vi "CSEI_log.vi"() -> ()   [LabVIEW 2010]
uses:
  <vilib>/Platform/TimedLoop/XDataNode/wakeup.ctl
  <vilib>/Platform/TimedLoop/XDataNode/XDNodeRunTimeDep.lvlib
  <vilib>/Platform/TimedLoop/XDataNode/nitl_modes.ctl
  <vilib>/Platform/TimedLoop/XDataNode/timing_clust.ctl
  <vilib>/Platform/TimedLoop/XDataNode/XDataNode.xnode
panel:
  out "Sample #":dbl
  out "Elapsed Time [s]":dbl
  out "Write to file":string
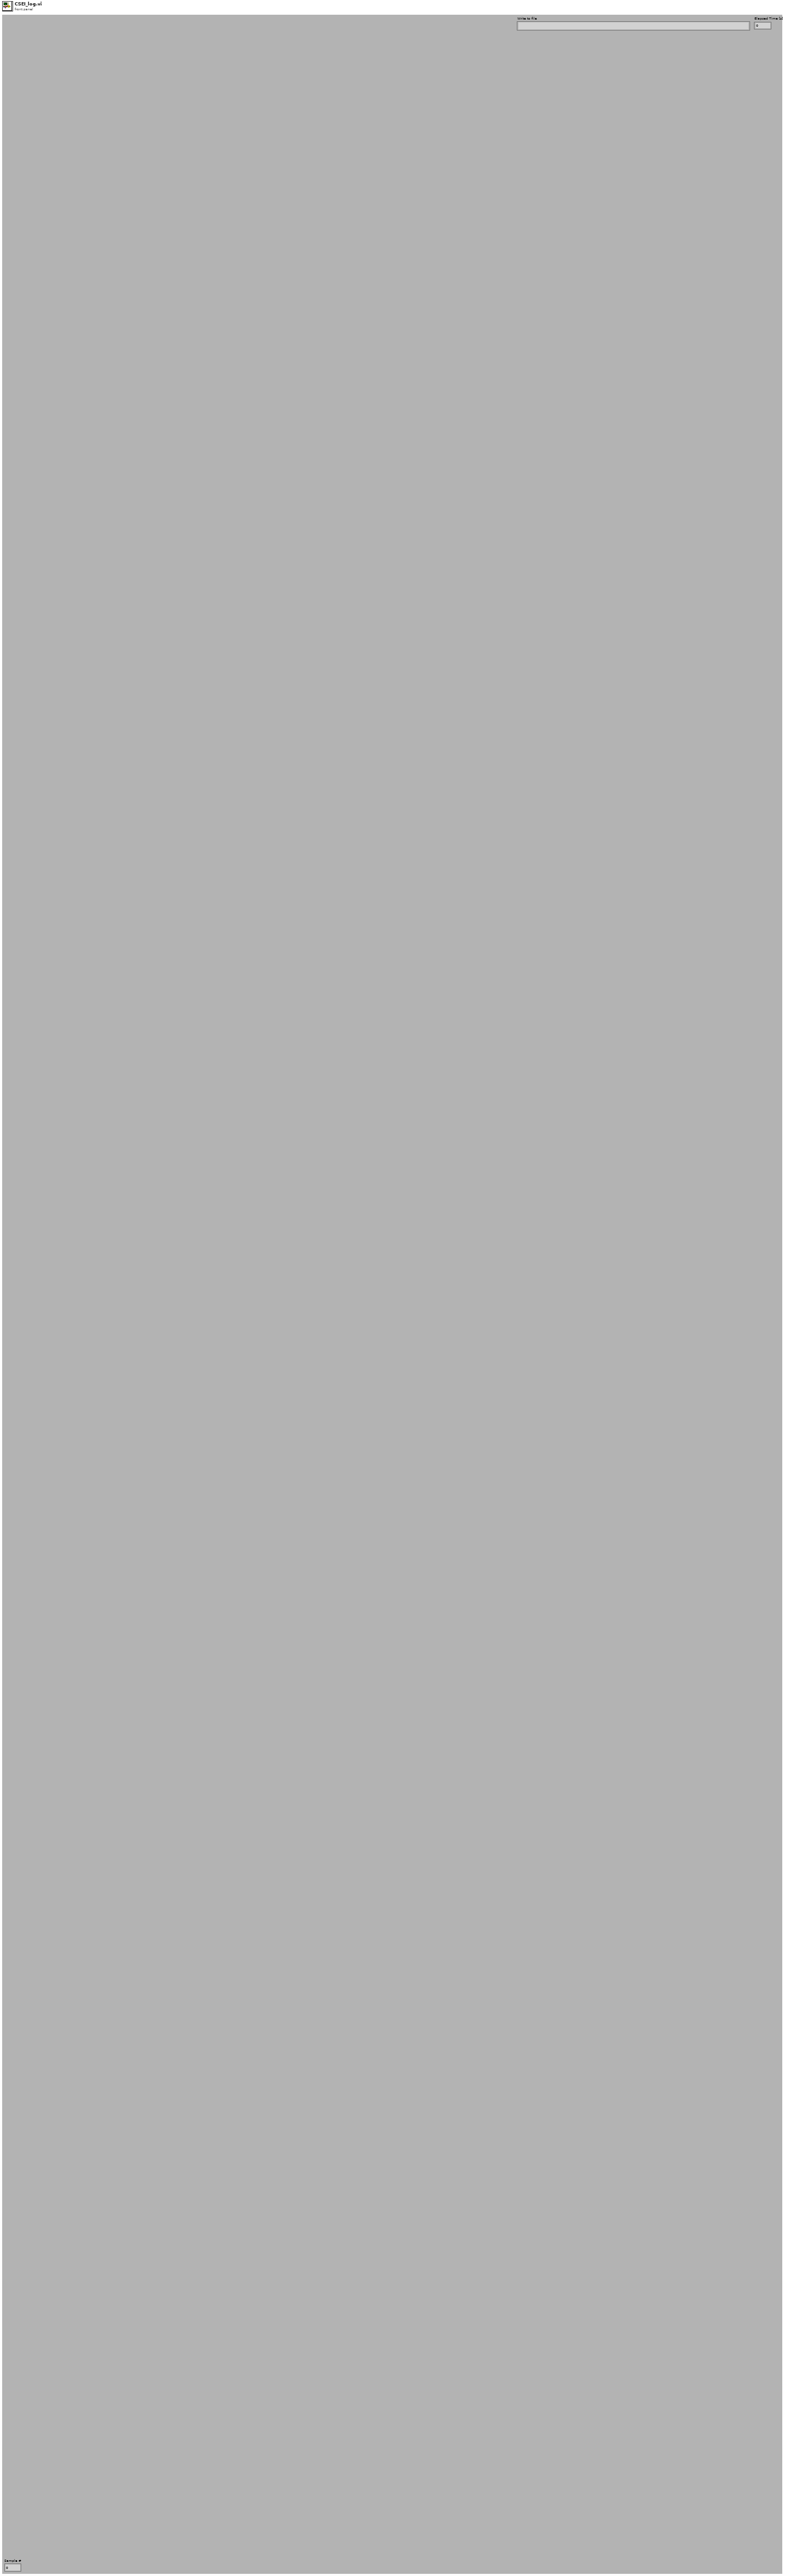
[diagram p1: front panel]
types:
  T1 = enum16{"open", "replace", "create", "open or create", "replace or create", "replace or create with confirmation"}
  T2 = typedef "XDNodeRunTimeDep.lvlib/timing_clust.ctl" = cluster{"Expected End [f-1]":u64, "Actual End [f-1]":u64, "Finished Late? [f-1]":bool, "Expected End [i-1]":u64, "Actual End [i-1]":u64, "Finished Late? [i-1]":bool, "Expected Start [i]":u64, "Actual Start [i]":u64, "Expected Start [f]":u64, "Actual Start [f]":u64, "Source Name":string, "Structure Name":string, "Period":i64, "Deadline":i64, "Offset":i64, "Start":i64, "Priority":i32, "Timeout":i32, "Mode":T3, "Wakeup Reason":T4, "Error":errorcluster, "Source Type":string, "Secondary Source Type":string, "Global End Time":u64, "Global Start Time":u64, "Frame Duration":u64, "Iteration Duration":u64, "Assigned CPU":i32, "I/O Scan Engine Mode":u32}
  T3 = typedef "XDNodeRunTimeDep.lvlib/nitl_modes.ctl" = enum32{"No Change", "Process missed periods, maintain original phase", "Discard missed periods, maintain original phase", "Process missed periods, ignore original phase", "Discard missed periods, ignore original phase"}
  T4 = typedef "XDNodeRunTimeDep.lvlib/wakeup.ctl" = enum32{"Normal", "Aborted", "Asynchronous wakeup", "Timing source error", "Timed loop error", "Timeout"}
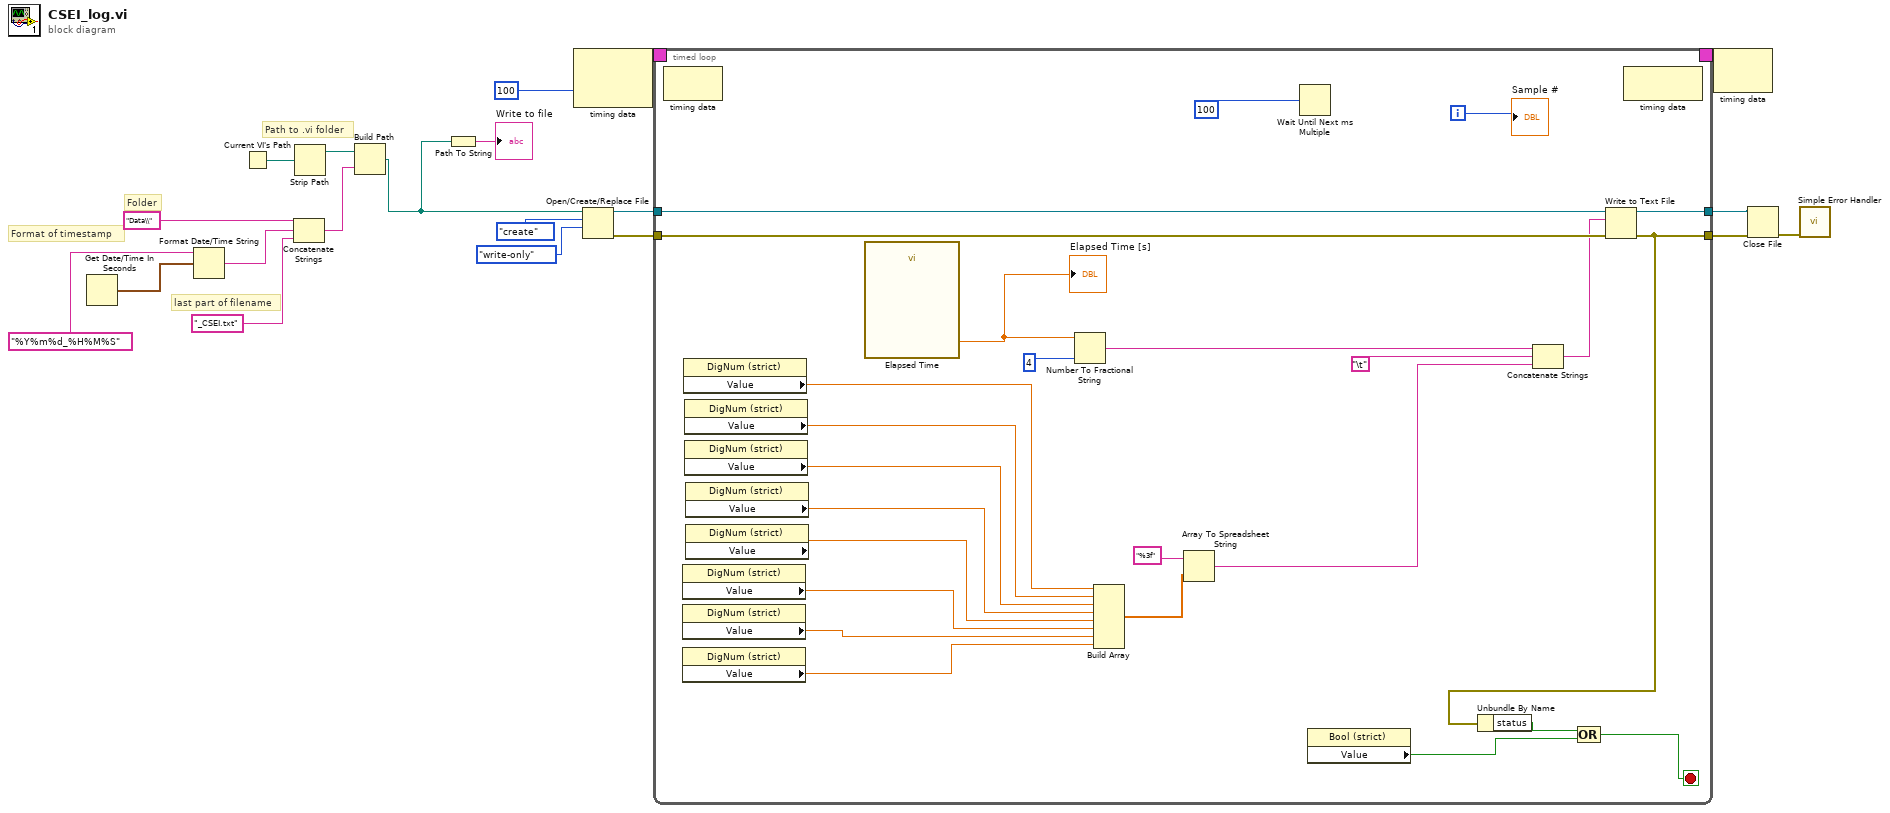
[diagram p0: block diagram]
diagram:
  # "Path to .vi folder"
  # "last part of filename"
  # "Folder"
  # "Format of timestamp"
  n1 = Get Date/Time In Seconds() -> (seconds since 1Jan1904=w17:timestamp)
  n2 = Format Date/Time String(time format string (%c)="%Y%m%d_%H%M%S", seconds (now)=w17) -> (date/time string=w15:string)  [unwired: 1 out]
  n3 = Current VI's Path() -> (path=w1:path)
  n4 = Concatenate Strings("Data\\" ("string"), w15, "_CSEI.txt" ("string")) -> (w12:string)
  n5 = Strip Path(path=w1) -> (stripped path=w14:path)  [unwired: 1 out]
  n6 = Build Path(base path=w14, name or relative path=w12) -> (appended path=w8:path)
  n7 = Path To String(path=w8) -> (string=→"Write to file":string)
  n8 = node-c288(100) -> (w20:T2)  [unwired: 1 in]
  n9 = Open/Create/Replace File(file path (use dialog)=w8, operation (0:open)=T1."create", access (0:read/write)=enum16{"read/write", "read-only", "write-only"}."write-only") -> (refnum out=w7:refnum<file>, error out=w5:errorcluster)  [unwired: 3 in, 1 out]
  n10 = timed-loop {
    timing: w20 -> [_]
    timing-out: [_] -> w19
    tunnel: w7 -> [w45]
    tunnel: [w44] -> w6
    tunnel: w5 -> [w43]
    tunnel: [w32] -> w4
    i -> [w38]
    stop <- w31 stop-if-true
    n11 = node-c288() -> ()  [unwired: 1 in, 1 out]
    n12 = property on="Property Node" class="DigNum (strict)"() -> ("Value"=w23:dbl)  [unwired: 2 in, 2 out]
    n13 = property on="Property Node" class="DigNum (strict)"() -> ("Value"=w22:dbl)  [unwired: 2 in, 2 out]
    n14 = property on="Property Node" class="DigNum (strict)"() -> ("Value"=w21:dbl)  [unwired: 2 in, 2 out]
    n15 = property on="Property Node" class="DigNum (strict)"() -> ("Value"=w28:dbl)  [unwired: 2 in, 2 out]
    n16 = property on="Property Node" class="DigNum (strict)"() -> ("Value"=w27:dbl)  [unwired: 2 in, 2 out]
    n17 = property on="Property Node" class="DigNum (strict)"() -> ("Value"=w26:dbl)  [unwired: 2 in, 2 out]
    n18 = property on="Property Node" class="DigNum (strict)"() -> ("Value"=w25:dbl)  [unwired: 2 in, 2 out]
    n19 = property on="Property Node" class="DigNum (strict)"() -> ("Value"=w24:dbl)  [unwired: 2 in, 2 out]
    n20 = call "Elapsed Time"() -> ("Elapsed Time (s)"=w33:dbl)  [unwired: 12 in, 7 out]
    "Elapsed Time [s]" <- w33
    n21 = Number To Fractional String(number=w33, precision (6)=4) -> (F-format string=w39:string)  [unwired: 2 in]
    n22 = Build Array(w28, w27, w26, w25, w24, w23, w22, w21) -> (w35:dbl[])
    n23 = Array To Spreadsheet String(array=w35, 3:"%3f") -> (spreadsheet string=w34:string)  [unwired: 1 in]
    n24 = Wait Until Next ms Multiple(millisecond multiple=100) -> ()  [unwired: 1 out]
    n25 = property on="Property Node" class="Bool (strict)"() -> ("Value"=w29:bool)  [unwired: 2 in, 2 out]
    n26 = Concatenate Strings(w39, "\t", w34) -> (w42:string)
    n27 = Write to Text File(file (use dialog)=w45, text=w42, error in=w43) -> (refnum out=w44:refnum<file>, error out=w32:errorcluster)  [unwired: 1 in, 1 out]
    n28 = Unbundle By Name(w32) -> ("status"=w30:bool)
    n29 = Compound Arithmetic op=OR(w30, w29) -> (w31:bool)
    n30 = node-c288() -> ()  [unwired: 1 in, 1 out]
    "Sample #" <- w38
  }
  n31 = node-c288(w19) -> ()  [unwired: 1 out]
  n32 = Close File(refnum=w6, error in=w4) -> (error out=w3:errorcluster)  [unwired: 1 out]
  n33 = call <vilib>:"Simple Error Handler.vi"("error in (no error)"=w3) -> ()  [unwired: 4 in, 5 out]
